vi "Import Custom Device Configuration.vi"(7 "Overwrite Existing?":bool=TRUE, 8 "error in (no error)":errorcluster, 9 "File Interface (.dat)":refnum<class "File Interface.lvclass">, 10 "Path":path, 11 "NodeID":u64) -> (0 "error out":errorcluster, 2 "cancelled":bool, 3 "NodeID out":u64)   [LabVIEW 2015, in "ImportExport.lvlib"]
doc: "ImportCDConfig.vi loads a configuration file (.dat) previously created using ExportCDConfig.vi. This configuration file includes the values for the properties of each Section, Channel, or Waveform in your Custom Device. It is strongly recommended to call this VI from your Initialization VI."
uses:
  ImportExport.lvlib
  File Interface Class/File Interface.lvclass
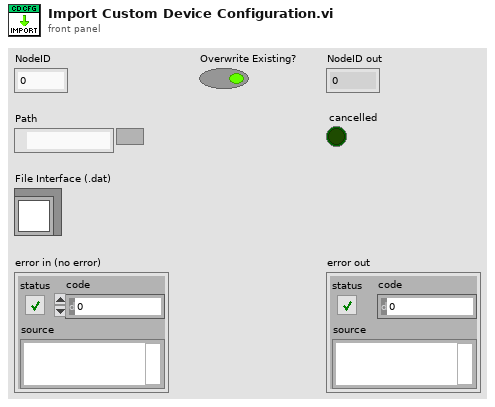
[diagram p1: front panel]
types:
  T1 = typedef "Advanced System Definition.lvlib/SysDef.Export.ctl" = cluster{"Version":string, "Tree":T2[]}
  T2 = typedef "Advanced System Definition.lvlib/TreeItem.ctl" = cluster{"Item Info":T3, "Parent Path":string[], "Properties":T8[]}
  T3 = typedef "Advanced System Definition.lvlib/TreeItem.Info.ctl" = cluster{"Name":string, "Description":string, "GUID":string, "Is Channel":bool, "Channel":T4, "Is Waveform":bool, "Waveform":T6}
  T4 = typedef "Custom Device API.lvlib/Custom Device Channel.ctl" = cluster{"Type":T5, "Units":string, "Default Value":dbl, "Faultable":bool, "Scalable":bool}
  T5 = typedef "Custom Device API.lvlib/Custom Device Channel Type.ctl" = enum16{"Input", "Output"}
  T6 = typedef "Custom Device API.lvlib/Custom Device Waveform.ctl" = cluster{"Data Type":T7, "Units":string}
  T7 = typedef "Custom Device API.lvlib/Custom Device Waveform DataType.ctl" = enum16{"Double", "Complex Double"}
  T8 = typedef "Advanced System Definition.lvlib/TreeItem.Property.ctl" = cluster{"Name":string, "Type":i32, "Value":variant}
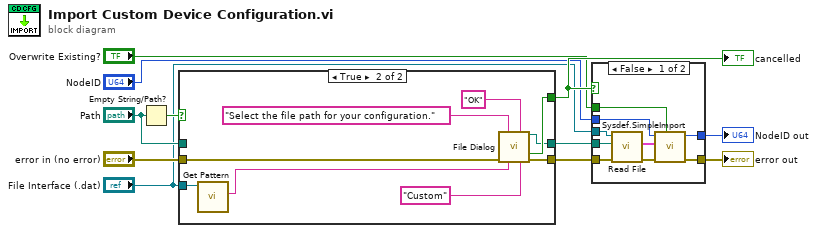
[diagram p0: block diagram]
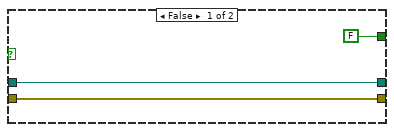
[diagram p2: hidden frame]
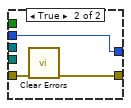
[diagram p3: hidden frame]
diagram:
  n1 = Empty String/Path?(string/path="Path") -> (empty?=w8:bool)
  n2 = case shown="True" w8 {
    tunnel: [FALSE ("cancelled") w20] -> w11
    tunnel: [w12 w19] -> w10
    tunnel: [w13 w18] -> w9
    tunnel: "error in (no error)" -> [w12 w17]
    tunnel: "Path" -> [w13 _]
    tunnel: "File Interface (.dat)" -> [_ w16]
    frame False {
    }
    frame True {
      n3 = call-dynamic "Get Pattern.vi"("File Interface in"=w16) -> ("file extension"=w15:string)  [unwired: 10 in]
      n4 = call "File Dialog"("prompt"="Select the file path for your configuration.", "button label"="OK", "error in"=w17, "pattern (all files)"=w15, "pattern label"="Custom") -> ("selected path"=w18:path, "cancelled"=w20:bool, "error out"=w19:errorcluster)  [unwired: 7 in, 1 out]
    }
  }
  "cancelled" <- w11
  n5 = case shown="False" w11 {
    tunnel: [w32 w34] -> w2
    tunnel: w10 -> [w25 w35]
    tunnel: w9 -> [w27 _]
    tunnel: "NodeID" -> [w31 w33]
    tunnel: [w30 w33] -> w4
    tunnel: "Overwrite Existing?" -> [w29 _]
    tunnel: "File Interface (.dat)" -> [w28 _]
    frame False {
      n6 = call-dynamic "Read File.vi"("error in (no error)"=w25, "Path in"=w27, "File Interface in"=w28) -> ("error out"=w26:errorcluster, "SysDef"=w24:T1)  [unwired: 7 in]
      n7 = call "Sysdef.SimpleImport.vi"("Overwrite Existing?"=w29, "error in (no error)"=w26, "SysDef"=w24, "NodeID"=w31) -> ("error out"=w32:errorcluster, "NodeID out"=w30:u64)  [unwired: 6 in]
    }
    frame True {
      n8 = call <vilib>:"Clear Errors.vi"("error in (no error)"=w35) -> ("error out"=w34:errorcluster)  [unwired: 5 in, 1 out]
    }
  }
  "error out" <- w2
  "NodeID out" <- w4
